vi "On Change Start Stop Camera Preview.vi"(8 "error in (no error)":errorcluster, 10 "Value":bool, 11 "App in":refnum<class "App.lvclass">) -> (0 "error out":errorcluster, 3 "App out":refnum<class "App.lvclass">)   [LabVIEW 2020, in "AR Example.lvlib" / "App.lvclass"]
uses:
  App.lvclass
  App.lvclass/App.ctl
  Timeout Action.ctl
  g_ar_toolkit.common/Image Size (Integer).ctl
  UI/UI.lvclass
  g_ar_toolkit.capture/CameraManager/CameraManager.lvclass
  g_ar_toolkit.capture/CameraStream/CameraStream.lvclass
  g_ar_toolkit.common/g_ar_toolkit.common.lvlib
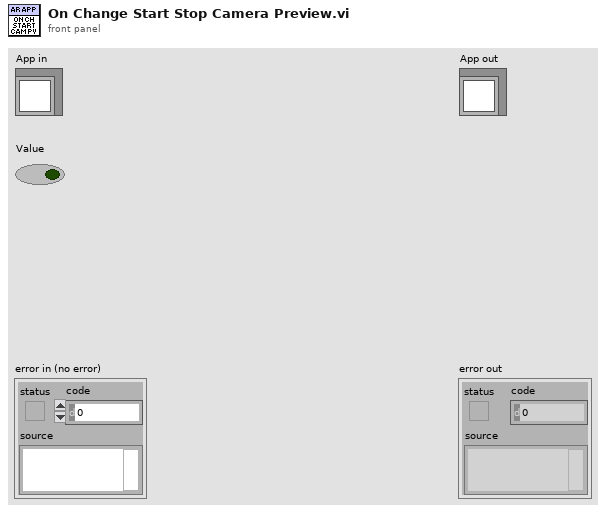
[diagram p1: front panel]
types:
  T1 = typedef "AR Example.lvlib/App.lvclass/Timeout Action.ctl" = enum16{"None", "Capture Preview Image"}
  T2 = typedef "g_ar_toolkit.common.lvlib/Image Size (Integer).ctl" = cluster{"Width":u16, "Height":u16}
  T3 = typedef "g_ar_toolkit.capture.lvlib/CameraManager.lvclass/Device Enumeration.ctl" = cluster{"Name":string, "Streams":set{T4}}
  T4 = typedef "g_ar_toolkit.capture.lvlib/CameraManager.lvclass/Stream Parameters.ctl" = cluster{"Width":u16, "Height":u16, "FPS":u8}
  T5 = typedef "g_ar_toolkit.image.lvlib/Image Draw Offset.ctl" = cluster{"Top":i16, "Left":i16}
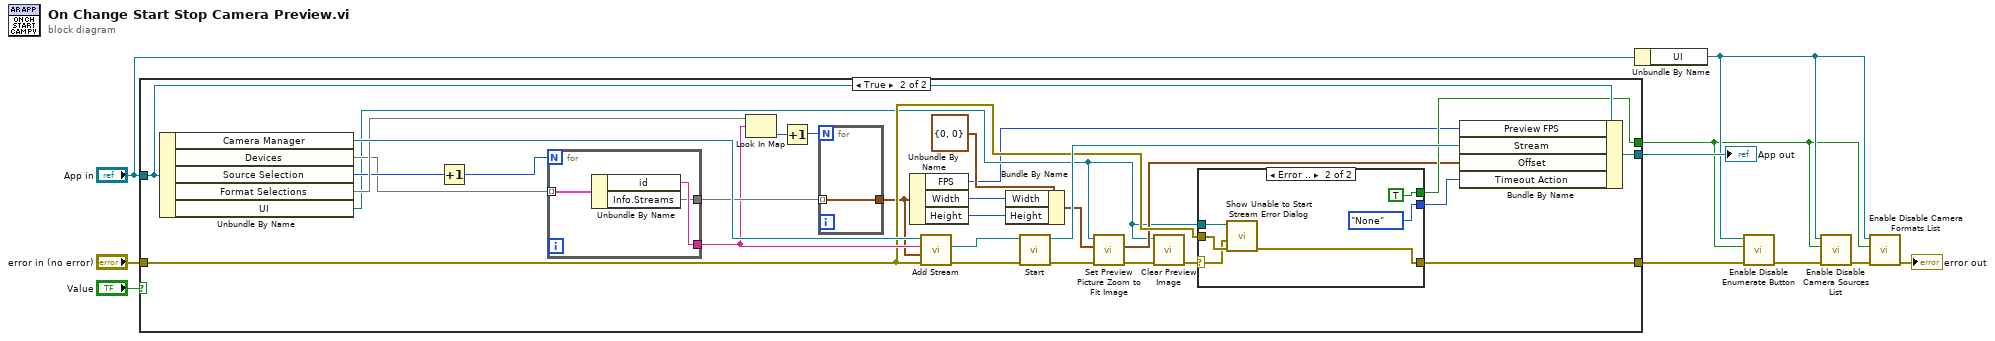
[diagram p0: block diagram]
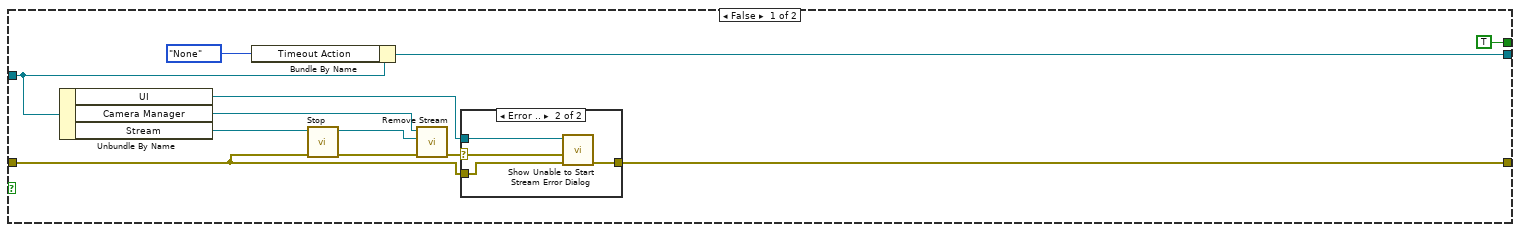
[diagram p2: hidden frame]
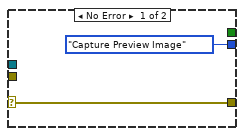
[diagram p4: hidden frame]
diagram:
  n1 = case shown="True" "Value" {
    tunnel: [w13 w42] -> w4
    tunnel: [w12 w43] -> w9
    tunnel: "App in" -> [w21 w56]
    tunnel: "error in (no error)" -> [w14 w41]
    tunnel: [TRUE w40] -> w5
    frame False {
      n2 = Unbundle By Name(w21) -> ("UI"=w17:refnum<class "UI.lvclass">, "Camera Manager"=w18:refnum<data-value>, "Stream"=w20:refnum<data-value>)
      n3 = Bundle By Name(cluster=w21, "Timeout Action"=Timeout_Action."None" ("Shared.Timeout Action")) -> (w12:refnum<class "App.lvclass">)
      n4 = call "Stop.vi"("error in (no error)"=w14, "Stream"=w20) -> ("error out"=w15:errorcluster, "Stream (duplicate)"=w19:refnum<data-value>)  [unwired: 8 in]
      n5 = call "Remove Stream.vi"("error in (no error)"=w15, "Stream"=w19, "CameraManager"=w18) -> ("error out"=w16:errorcluster)  [unwired: 7 in, 1 out]
      n6 = case shown="Error .." w16 {
        selector: w16 -> [w23 w26]
        tunnel: w17 -> [_ w27]
        tunnel: w14 -> [_ w25]
        tunnel: [w23 w24] -> w13
        frame No Error {
        }
        frame Error {
          n7 = call-dynamic "Show Unable to Start Stream Error Dialog.vi"("error in (no error)"=w25, "Stream Start Error"=w26, "UI in"=w27) -> ("error out"=w24:errorcluster)  [unwired: 8 in]
        }
      }
    }
    frame True {
      n8 = Unbundle By Name(w56) -> ("Camera Manager"=w55:refnum<data-value>, "Devices"=w49:map{string, T3}, "Source Selection"=w51:i32, "Format Selections"=w54:map{string, i32}, "UI"=w29:refnum<class "UI.lvclass">)
      n9 = Increment(x=w51) -> (x+1=w50:i32)
      n10 = for {
        N: w50 -> [_]
        tunnel: w49 -> [w67] mode=indexing
        tunnel: [w66] -> w47
        tunnel: [w65] -> w48
        n11 = Unbundle By Name(w67) -> ("id"=w66:string, "Info.Streams"=w65:set{T4})
      }
      n12 = Look In Map(map=w54, key=w47) -> (value=w53:i32)  [unwired: 1 in, 1 out]
      n13 = Increment(x=w53) -> (x+1=w52:i32)
      n14 = for {
        N: w52 -> [_]
        tunnel: w48 -> [w68] mode=indexing
        tunnel: [w68] -> w39
      }
      n15 = Unbundle By Name(w39) -> ("FPS"=w28:u8, "Width"=w36:u16, "Height"=w35:u16)
      n16 = call "Add Stream.vi"("error in (no error)"=w41, "Desired Stream Parameters"=w39, "Device ID"=w47, "CameraManager"=w55) -> ("error out"=w46:errorcluster, "Stream"=w45:refnum<data-value>)  [unwired: 5 in, 1 out]
      n17 = Bundle By Name(cluster=T2 {"Width"=0, "Height"=0} ("Size"), "Width"=w36, "Height"=w35) -> (w37:T2)
      n18 = call "Start.vi"("error in (no error)"=w46, "Stream"=w45) -> ("error out"=w34:errorcluster, "Stream (duplicate)"=w44:refnum<data-value>)  [unwired: 8 in]
      n19 = call-dynamic "Set Preview Picture Zoom to Fit Image.vi"("error in (no error)"=w34, "Size"=w37, "UI in"=w29) -> ("error out"=w33:errorcluster, "Offset"=w32:T5)  [unwired: 7 in]
      n20 = call-dynamic "Clear Preview Image.vi"("error in (no error)"=w33, "UI in"=w29) -> ("error out"=w30:errorcluster)  [unwired: 9 in]
      n21 = case shown="Error .." w30 {
        selector: w30 -> [w58 w62]
        tunnel: [w58 w63] -> w42
        tunnel: w41 -> [_ w64]
        tunnel: [Timeout_Action."Capture Preview Image" ("Shared.Timeout Action") Timeout_Action."None" ("Shared.Timeout Action")] -> w31
        tunnel: [_ TRUE] -> w40
        tunnel: w29 -> [_ w59]
        frame No Error {
        }
        frame Error {
          n22 = call-dynamic "Show Unable to Start Stream Error Dialog.vi"("error in (no error)"=w64, "Stream Start Error"=w62, "UI in"=w59) -> ("error out"=w63:errorcluster)  [unwired: 8 in]
        }
      }
      n23 = Bundle By Name(cluster=w56, "Preview FPS"=w28, "Stream"=w44, "Offset"=w32, "Timeout Action"=w31) -> (w43:refnum<class "App.lvclass">)
    }
  }
  "App out" <- w9
  n24 = Unbundle By Name("App in") -> ("UI"=w6:refnum<class "UI.lvclass">)
  n25 = call-dynamic "Enable Disable Enumerate Button.vi"("error in (no error)"=w4, "Enable?"=w5, "UI in"=w6) -> ("error out"=w3:errorcluster)  [unwired: 8 in]
  n26 = call-dynamic "Enable Disable Camera Sources List.vi"("error in (no error)"=w3, "Enable?"=w5, "UI in"=w6) -> ("error out"=w2:errorcluster)  [unwired: 8 in]
  n27 = call-dynamic "Enable Disable Camera Formats List.vi"("error in (no error)"=w2, "Enable?"=w5, "UI in"=w6) -> ("error out"=→"error out":errorcluster)  [unwired: 8 in]
